vi "Live_Example_IMAQ.vi"() -> ()   [LabVIEW 2019]
doc: "This example demonstrates the image acquisition with one camera in ring buffer mode together with a live display of the latest images during record. After record is stopped, the images can be addressed by index.\nNote that this example will not be fail save, i.e. doesnt react on errors, just handles them forward to the end\n\nUsage:\nSelect your required image count, data format and the camera setup before you start the program.\nOnce started, the camera class will be initialized and images will be recorded and displayed automatically\nYou can stop the images by pressing stop record.\nAfter stopped, the image at the selected index will be read out\nTo finish the program click on quit application, this will force an exit of the camera class\nYou can change your required ROI after and also during the record."
uses:
  camera/Camera.lvclass
  pco.sdk/TimingControl/TimingControl.lvlib
panel:
  in  "Trigger":bool
  in  "data_format":T1(ring)=enum."Mono16"
  out "Image":T2(plugin-control)
  out "rawImage":u16[][](array[numeric])
  in  "Image Index":u32 max=9
  out "Recorded Images":u32
  in  "TriggerMode":T3(ring)
  in  "Quit":bool
  out "Error":errorcluster {"code" format="%x"}
  in  "Stop Record":bool
  out "Recording On":bool
  in  "cropY1":u64=2 min=1 max=1040 step=1
  in  "cropX1":u64=2 min=1 max=1392 step=1
  in  "cropY0":u64=1 min=1 max=1039 step=1
  in  "cropX0":u64=1 min=1 max=1391 step=1
  out "Image Height":u64
  out "Image Width":u64
  in  "dwImgCount":u32=10 caption="Required Number of Images" max=2397
  in  "Exposure Time [s]":dbl=0.010000000000000002 min=1e-06 max=60.0 step=0.001
  # "This example demonstrates the image acquisition with one camera in ring buffer mode together with a live display of the latest images during record. After record is stopped, the images can be addressed by index.\nNote that this example will not be fail save, i.e. doesnt react on errors, just handles them forward to the end\n\nUsage:\nSelect your required image count, data format and the camera setup before you start the program.\nOnce started, the camera class will be initialized and images will be recorded and displayed automatically\nYou can stop the images by pressing stop record.\nAfter stopped, the image at the selected index will be read out\nTo finish the program click on quit application, this will force an exit of the camera class\nYou can change the cropped region during or after recording."
  # "pco.labview"
  # "Camera Setup"
  # "Recording Control"
  # "Parameters for image readout"
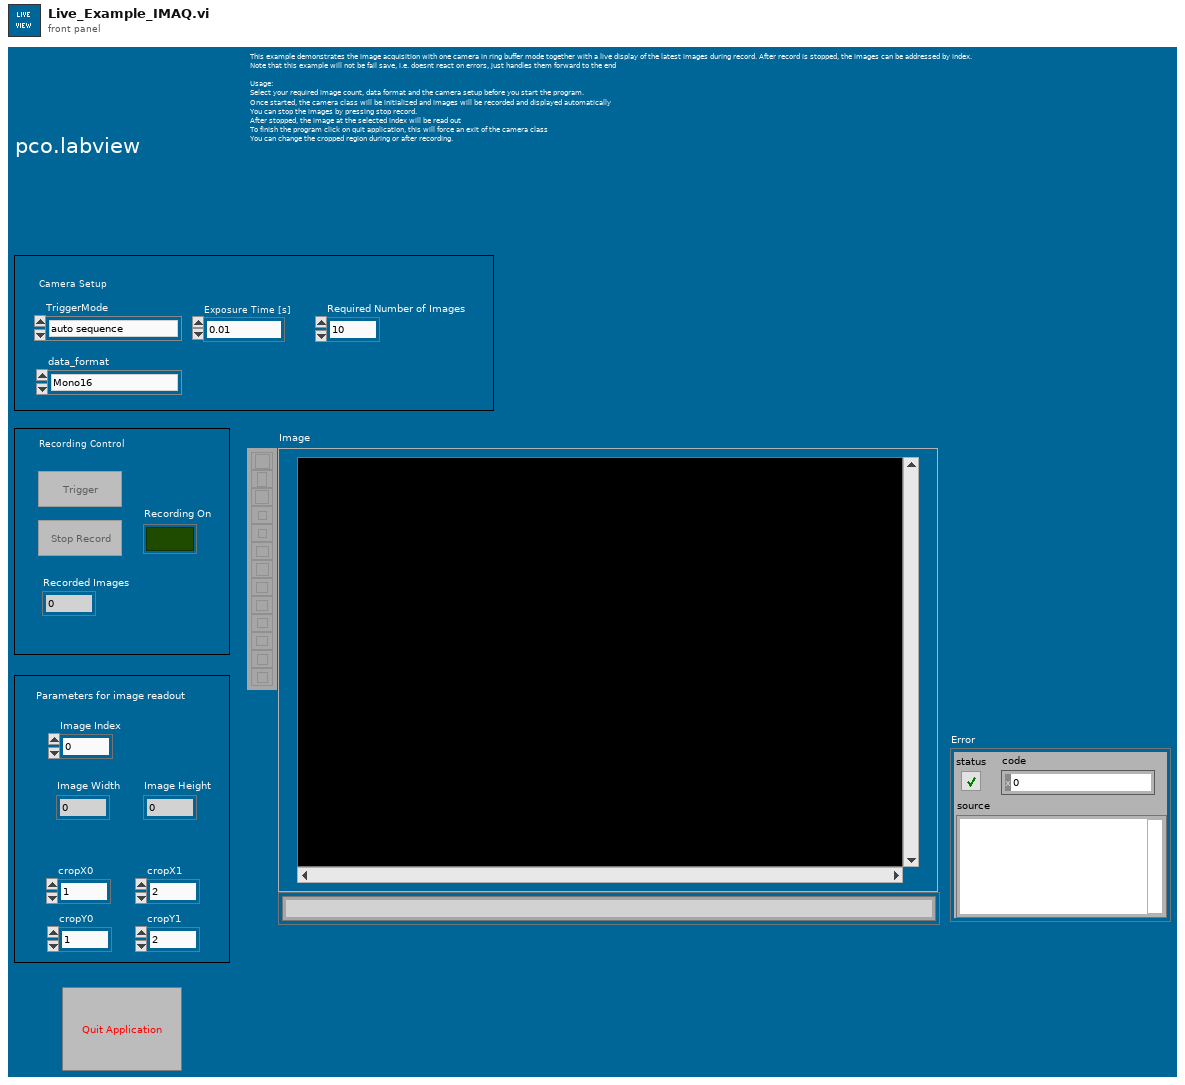
[diagram p1: front panel]
types:
  T1 = enum16{"Undefined", "Mono8", "Mono16", "BGRA8", "RGBA8", "BGRA16", "RGBA16", "CompressedMono8"}
  T2 = typedef "IMAQ Image.ctl" = refnum<image>
  T3 = enum16{"auto sequence", "software trigger", "external exposure start", "external exposure control"}
  T4 = enum16{"sequence", "sequence non blocking", "ring buffer", "fifo", "tif", "multitif", "pcoraw", "b16", "dicom", "multidicom", "camram_ring", "camram_segment"}
  T5 = enum8{"Enabled", "Disabled", "Disabled and Grayed Out"}
  T6 = cluster{"serial":u32, "type":u16, "sub_type":u16, "interface_type":u16, "bit_resolution":u16, "min_exposure_time_s":dbl, "max_exposure_time_s":dbl, "min_exposure_step_s":dbl, "min_delay_time_s":dbl, "max_delay_time_s":dbl, "min_delay_step_s":dbl, "min_width":u64, "min_height":u64, "max_width":u64, "max_height":u64, "roi_step_horz":u64, "roi_step_vert":u64, "roi_symmetric_horz":bool, "roi_symmetric_vert":bool, "has_timestamp_mode":bool, "has_timestamp_mode_ascii_only":bool, "pixelrate_vec":u32[], "conversion_factor_vec":sgl[], "has_trigger_mode_extexpctrl":bool, "has_acquire_mode":bool, "has_ext_acquire_mode":bool, "has_metadata_mode":bool, "has_ram":bool, "binning_horz_vec":u16[], "binning_vert_vec":u16[], "has_average_binning":bool, "pixel_format_vec":u32[]}
  T7 = typedef "Image Type" = u32
  T8 = cluster{"wSignalNum":u16, "wEnabled":u16, "wType":u16, "wPolarity":u16, "wFilterSetting":u16, "wSelected":u16, "dwParameter":u32[], "dwSignalFunctionality":u32[]}
  T9 = typedef "Camera.lvclass/binning.ctl" = cluster{"vert":u16, "horz":u16, "mode":u16}
  T10 = cluster{"exposure_time_s":dbl, "delay_time_s":dbl, "roi":cluster{"x0":u64, "y0":u64, "x1":u64, "y1":u64}, "timestamp_mode":u16, "pixelrate":u32, "conversion_factor":sgl, "trigger_mode":u16, "acquire_mode":u16, "acquire_sequence_number":u32, "metadata_mode":u16, "noisefilter_mode":u16, "pixel_format":u32, "binning":T9, "auto_exposure":cluster{"region":u16, "min_exposure_s":dbl, "max_exposure_s":dbl}}
  T11 = cluster{"Plane 4 (alpha)":u16, "Plane 1 (Red)":u16, "Plane 2 (Green)":u16, "Plane 3 (Blue)":u16}[][]
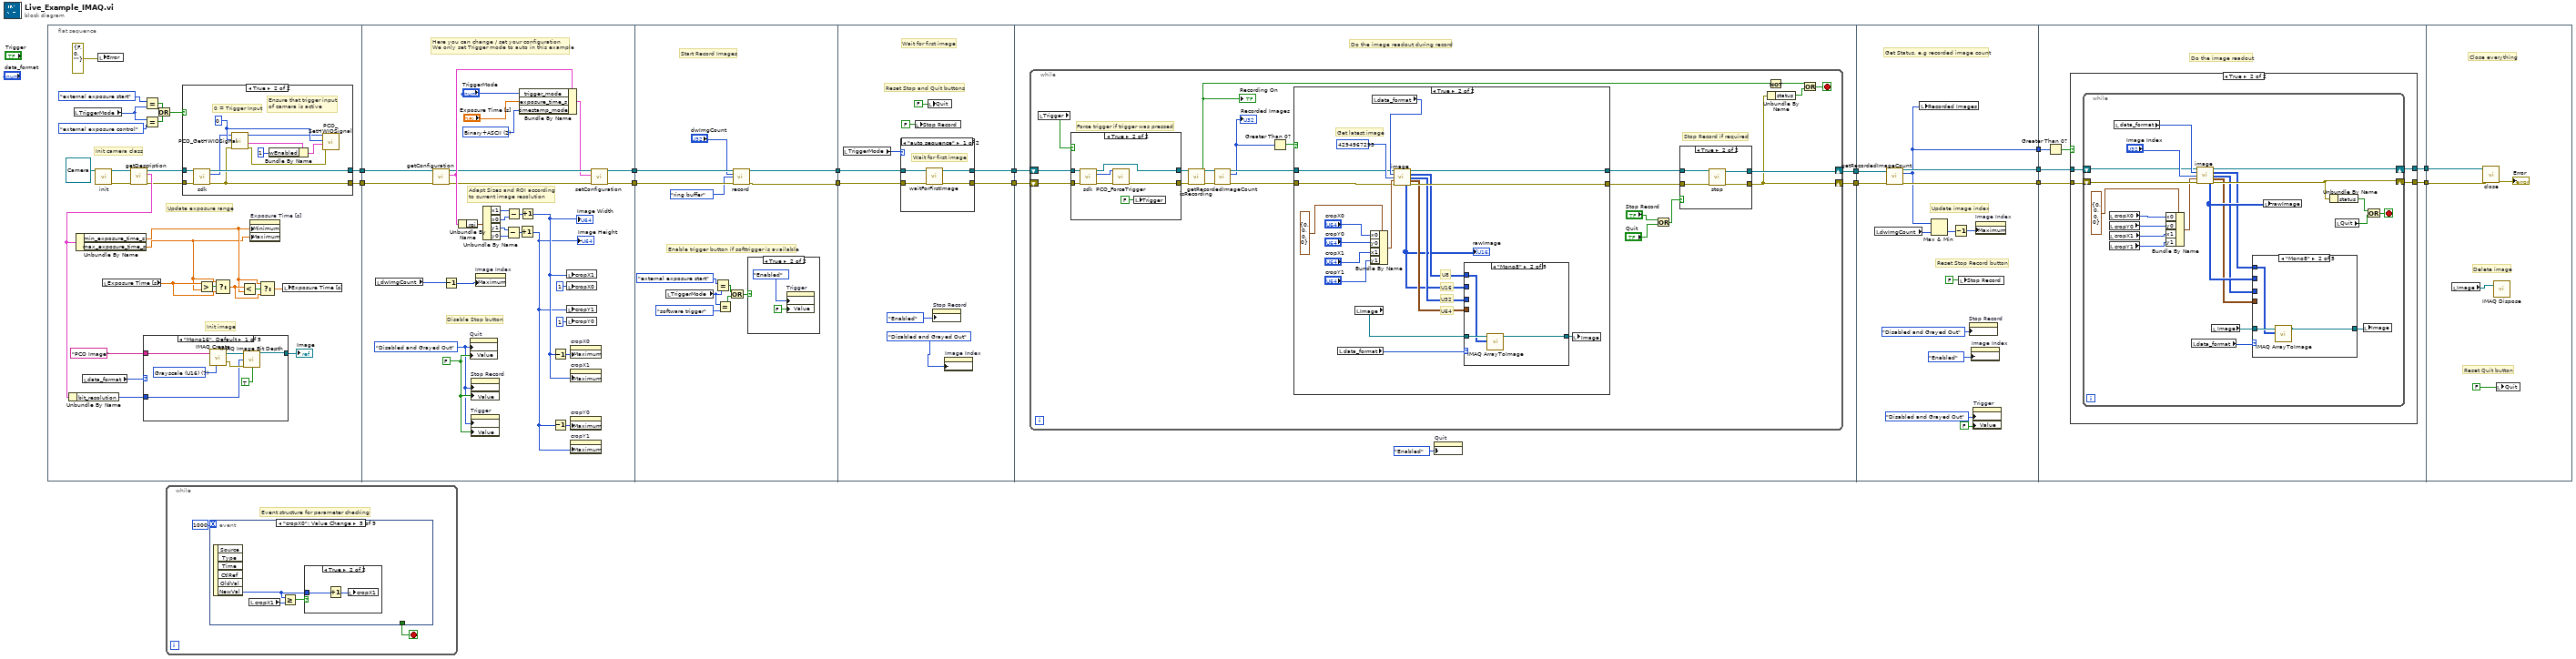
[diagram p0: block diagram]
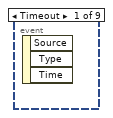
[diagram p2: hidden frame]
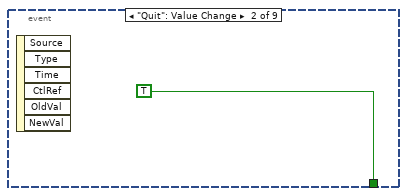
[diagram p3: hidden frame]
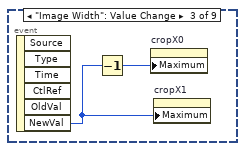
[diagram p4: hidden frame]
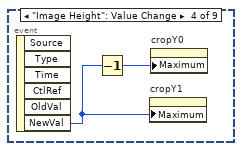
[diagram p5: hidden frame]
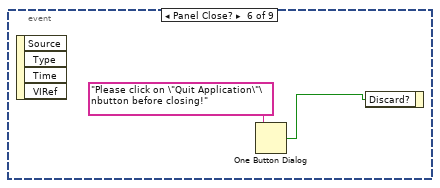
[diagram p7: hidden frame]
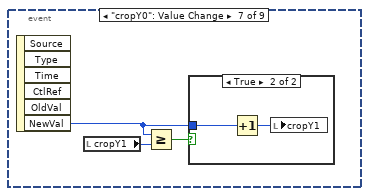
[diagram p8: hidden frame]
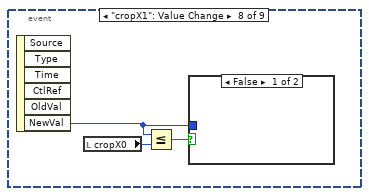
[diagram p10: hidden frame]
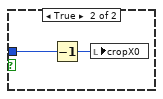
[diagram p11: hidden frame]
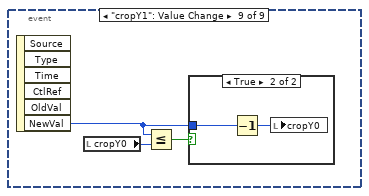
[diagram p12: hidden frame]
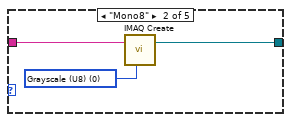
[diagram p15: hidden frame]
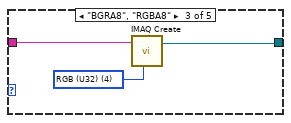
[diagram p16: hidden frame]
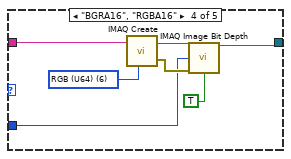
[diagram p17: hidden frame]
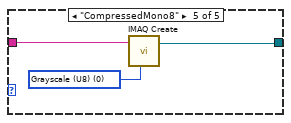
[diagram p18: hidden frame]
diagram:
  n1 = flat-sequence {
    tunnel: [w23] -> w7
    tunnel: [w22] -> w6
    tunnel: [w82] -> w15
    tunnel: [w86] -> w14
    tunnel: w7 -> [w81]
    tunnel: w6 -> [w80]
    tunnel: [w107] -> w9
    tunnel: [w108] -> w8
    tunnel: w14 -> [w117]
    tunnel: w15 -> [w116]
    tunnel: w9 -> [w124]
    tunnel: w8 -> [w125]
    tunnel: [w123] -> w13
    tunnel: [w121] -> w2
    tunnel: w13 -> [w139]
    tunnel: [w137] -> w12
    tunnel: [w136] -> w5
    tunnel: w2 -> [w135]
    tunnel: w12 -> [w222]
    tunnel: [w220] -> w11
    tunnel: w5 -> [w215]
    tunnel: [w214] -> w4
    tunnel: [w213] -> w1
    tunnel: w11 -> [w231]
    tunnel: [w230] -> w10
    tunnel: w4 -> [w229]
    tunnel: [w228] -> w3
    tunnel: w1 -> [w226]
    tunnel: w10 -> [w278]
    tunnel: w3 -> [w276]
    frame #0 {
      # "Init image"
      # "Init camera class"
      # "Update exposure range"
      n2 = local read "TriggerMode"() -> (w17:T3)
      n3 = local read "data_format"() -> (w28:T1)
      n4 = call-dynamic "init.vi"("Camera in"=refnum<class "Camera.lvclass"> refnum) -> ("Camera out"=w31:refnum<class "Camera.lvclass">, "error out"=w32:errorcluster)  [unwired: 8 in]
      n5 = local write "Error"(errorcluster {"status"=FALSE, "code"=0, "source"=""} ("error IO")) -> ()
      n6 = local read "Exposure Time [s]"() -> (w40:dbl)
      n7 = call-dynamic "getDescription.vi"("error in (no error)"=w32, "Camera in"=w31) -> ("error out"=w24:errorcluster, "description"=w27:T6, "Camera out"=w25:refnum<class "Camera.lvclass">)  [unwired: 7 in]
      n8 = Unbundle By Name(w27) -> ("bit_resolution"=w26:u16)
      n9 = Unbundle By Name(w27) -> ("min_exposure_time_s"=w30:dbl, "max_exposure_time_s"=w29:dbl)
      n10 = case shown="\"Mono16\", Default" w28 {
        tunnel: "PCO Image" ("Image Name") -> [w60 w64 w66 w73 w76]
        tunnel: [w56 w62 w65 w70 w75] -> w33
        tunnel: w26 -> [w55 _ _ w68 _]
        frame "Mono16", Default {
          w61 = T7 7 items=["Grayscale (U8)", "Grayscale (I16)", "Grayscale (SGL)", "Complex (CSG)", "RGB (U32)", "HSL (U32)", "RGB (U64)", "Grayscale (U16)"] ("Image Type")
          n11 = call "IMAQ Create"("Image Name"=w60, "Image Type"=w61) -> ("New Image"=w58:T2, "error out"=w57:errorcluster)  [unwired: 3 in]
          n12 = call "IMAQ Image Bit Depth"("Image"=w58, "Bit Depth (0)"=w55, "error in (no error)"=w57, "Get/Set Bit Depth? (Set)"=TRUE) -> ("Image Out"=w56:T2)  [unwired: 9 in, 2 out]
        }
        frame "Mono8" {
          w63 = T7 0 items=["Grayscale (U8)", "Grayscale (I16)", "Grayscale (SGL)", "Complex (CSG)", "RGB (U32)", "HSL (U32)", "RGB (U64)", "Grayscale (U16)"] ("Image Type")
          n13 = call "IMAQ Create"("Image Name"=w64, "Image Type"=w63) -> ("New Image"=w62:T2)  [unwired: 3 in, 1 out]
        }
        frame "BGRA8", "RGBA8" {
          w67 = T7 4 items=["Grayscale (U8)", "Grayscale (I16)", "Grayscale (SGL)", "Complex (CSG)", "RGB (U32)", "HSL (U32)", "RGB (U64)", "Grayscale (U16)"] ("Image Type")
          n14 = call "IMAQ Create"("Image Name"=w66, "Image Type"=w67) -> ("New Image"=w65:T2)  [unwired: 3 in, 1 out]
        }
        frame "BGRA16", "RGBA16" {
          w74 = T7 6 items=["Grayscale (U8)", "Grayscale (I16)", "Grayscale (SGL)", "Complex (CSG)", "RGB (U32)", "HSL (U32)", "RGB (U64)", "Grayscale (U16)"] ("Image Type")
          n15 = call "IMAQ Create"("Image Name"=w73, "Image Type"=w74) -> ("New Image"=w71:T2, "error out"=w69:errorcluster)  [unwired: 3 in]
          n16 = call "IMAQ Image Bit Depth"("Image"=w71, "Bit Depth (0)"=w68, "error in (no error)"=w69, "Get/Set Bit Depth? (Set)"=TRUE) -> ("Image Out"=w70:T2)  [unwired: 9 in, 2 out]
        }
        frame "CompressedMono8" {
          w77 = T7 0 items=["Grayscale (U8)", "Grayscale (I16)", "Grayscale (SGL)", "Complex (CSG)", "RGB (U32)", "HSL (U32)", "RGB (U64)", "Grayscale (U16)"] ("Image Type")
          n17 = call "IMAQ Create"("Image Name"=w76, "Image Type"=w77) -> ("New Image"=w75:T2)  [unwired: 3 in, 1 out]
        }
      }
      "Image" <- w33
      n18 = Equal?(x=T3."external exposure start" ("TriggerMode"), y=w17) -> (x = y?=w20:bool)
      n19 = Equal?(x=w17, y=T3."external exposure control" ("TriggerMode")) -> (x = y?=w19:bool)
      n20 = Or(x=w20, y=w19) -> (x .or. y?=w18:bool)
      n21 = case shown="True" w18 {
        tunnel: w25 -> [w43 w48]
        tunnel: w24 -> [w42 w47]
        tunnel: [w43 w46] -> w23
        tunnel: [w42 w44] -> w22
        frame False {
        }
        frame True {
          w52 = u16 0 ("wSignalNum")
          # "0 = Trigger Input"
          # "Ensure that trigger input\nof camera is active"
          n22 = call-dynamic "sdk.vi"("Camera in"=w48, "error in (no error)"=w47) -> ("Camera out"=w46:refnum<class "Camera.lvclass">, "sdk"=w45:u64, "error out"=w44:errorcluster)  [unwired: 11 in]
          n23 = call "PCO_GetHWIOSignal.vi"("error in (no error)"=w44, "wSignalNum"=w52, "ph"=w45) -> ("error out"=w50:errorcluster, "strSignal"=w54:T8, "ph out"=w49:u64)  [unwired: 5 in, 1 out]
          n24 = Bundle By Name(cluster=w54, "wEnabled"=u16 1) -> (w51:T8)
          n25 = call "PCO_SetHWIOSignal.vi"("error in (no error)"=w50, "strSignal"=w51, "wSignalNum"=w52, "ph"=w49) -> ()  [unwired: 5 in, 3 out]
        }
      }
      n26 = Greater?(x=w40, y=w29) -> (0:w41:bool)
      n27 = Select(t=w29, s=w41, f=w40) -> (s? t:f=w38:dbl)
      n28 = Less?(x=w38, y=w30) -> (x < y?=w39:bool)
      n29 = property on="Exposure Time [s]" class="DigNum (strict)"("Minimum"=w30, "Maximum"=w29) -> ()  [unwired: 2 in, 2 out]
      n30 = Select(t=w30, s=w39, f=w38) -> (s? t:f=w37:dbl)
      n31 = local write "Exposure Time [s]"(w37) -> ()
    }
    frame #1 {
      w92 = u16 2 items=["OFF", "Binary", "Binary+ASCII", "ASCII"] ("wTimeStampMode")
      w79 = FALSE ("Stop")
      w78 = T5."Disabled and Grayed Out" ("Disabled")
      # "Disable Stop button"
      # "Adapt Sizes and ROI according\nto current image resolution"
      # "Here you can change / set your configuration\nWe only set Trigger mode to auto in this example"
      n32 = local read "dwImgCount"() -> (w93:u32)
      n33 = call-dynamic "getConfiguration.vi"("error in (no error)"=w80, "Camera in"=w81) -> ("error out"=w87:errorcluster, "configuration"=w98:T10, "Camera out"=w89:refnum<class "Camera.lvclass">)  [unwired: 7 in]
      n34 = Decrement(x=w93) -> (x-1=w83:u32)
      n35 = Unbundle By Name(w98) -> ("roi"=w99:cluster{"x0":u64, "y0":u64, "x1":u64, "y1":u64})
      n36 = property on="Quit" class="Bool (strict)"("DisabledEnum"=w78, "Value"=w79) -> ()  [unwired: 2 in, 2 out]
      n37 = property on="Stop Record" class="Bool (strict)"("DisabledEnum"=w78, "Value"=w79) -> ()  [unwired: 2 in, 2 out]
      n38 = property on="Trigger" class="Bool (strict)"("DisabledEnum"=w78, "Value"=w79) -> ()  [unwired: 2 in, 2 out]
      n39 = property on="Image Index" class="DigNum (strict)"("Maximum"=w83) -> ()  [unwired: 2 in, 2 out]
      n40 = Unbundle By Name(w99) -> ("x1"=w101:u64, "x0"=w100:u64, "y1"=w103:u64, "y0"=w102:u64)
      n41 = Subtract(x=w103, y=w102) -> (x-y=w105:u64)
      n42 = Subtract(x=w101, y=w100) -> (x-y=w104:u64)
      n43 = Bundle By Name(cluster=w98, "trigger_mode"="TriggerMode", "exposure_time_s"="Exposure Time [s]", "timestamp_mode"=w92) -> (w88:T10)
      n44 = Increment(x=w105) -> (x+1=w84:u64)
      "Image Height" <- w84
      n45 = Increment(x=w104) -> (x+1=w85:u64)
      "Image Width" <- w85
      n46 = Decrement(x=w85) -> (x-1=w96:u64)
      n47 = Decrement(x=w84) -> (x-1=w97:u64)
      n48 = local write "cropX1"(w85) -> ()
      n49 = local write "cropX0"(u64 1 ("roiY0")) -> ()
      n50 = local write "cropY1"(w84) -> ()
      n51 = local write "cropY0"(u64 1 ("roiY0")) -> ()
      n52 = property on="cropX0" class="DigNum (strict)"("Maximum"=w96) -> ()  [unwired: 2 in, 2 out]
      n53 = property on="cropX1" class="DigNum (strict)"("Maximum"=w85) -> ()  [unwired: 2 in, 2 out]
      n54 = property on="cropY0" class="DigNum (strict)"("Maximum"=w97) -> ()  [unwired: 2 in, 2 out]
      n55 = property on="cropY1" class="DigNum (strict)"("Maximum"=w84) -> ()  [unwired: 2 in, 2 out]
      n56 = call-dynamic "setConfiguration.vi"("error in (no error)"=w87, "configuration"=w88, "Camera in"=w89) -> ("error out"=w86:errorcluster, "Camera out"=w82:refnum<class "Camera.lvclass">)  [unwired: 7 in]
    }
    frame #2 {
      # "Enable trigger button if softtrigger is available"
      # "Start Record Images"
      n57 = local read "TriggerMode"() -> (w113:T3)
      n58 = Equal?(x=T3."external exposure start" ("TriggerMode"), y=w113) -> (x = y?=w110:bool)
      n59 = Equal?(x=w113, y=T3."software trigger" ("TriggerMode")) -> (x = y?=w109:bool)
      n60 = Or(x=w110, y=w109) -> (x .or. y?=w111:bool)
      n61 = call-dynamic "record.vi"("Camera in"=w116, "num_images"="dwImgCount", "record_mode"=T4."ring buffer", "error in (no error)"=w117) -> ("Camera out"=w108:refnum<class "Camera.lvclass">, "error out"=w107:errorcluster)  [unwired: 10 in]
      n62 = case shown="True" w111 {
        frame False {
        }
        frame True {
          n63 = property on="Trigger" class="Bool (strict)"("DisabledEnum"=T5."Enabled" ("Disabled"), "Value"=FALSE ("Trigger")) -> ()  [unwired: 2 in, 2 out]
        }
      }
    }
    frame #3 {
      # "Wait for first image"
      # "Reset Stop and Quit buttons"
      n64 = local read "TriggerMode"() -> (w120:T3)
      n65 = case shown="\"auto sequence\"" w120 {
        tunnel: w125 -> [w132 w134]
        tunnel: w124 -> [w131 w133]
        tunnel: [w130 w133] -> w123
        tunnel: [w129 w134] -> w121
        frame "auto sequence" {
          # "Wait for first image"
          n66 = call-dynamic "waitForFirstImage.vi"("error in (no error)"=w131, "Camera in"=w132) -> ("error out"=w130:errorcluster, "Camera out"=w129:refnum<class "Camera.lvclass">)  [unwired: 8 in]
        }
        frame Default {
        }
      }
      n67 = local write "Stop Record"(FALSE ("Stop Record")) -> ()
      n68 = local write "Quit"(FALSE ("Stop")) -> ()
      n69 = property on="Stop Record" class="Bool (strict)"("DisabledEnum"=T5."Enabled" ("Disabled")) -> ()  [unwired: 2 in, 2 out]
      n70 = property on="Image Index" class="DigNum (strict)"("DisabledEnum"=T5."Disabled and Grayed Out" ("Disabled")) -> ()  [unwired: 2 in, 2 out]
    }
    frame #4 {
      # "Do the image readout during record"
      n71 = while {
        shift-right: [w142] -> w137
        shift-left: w139 -> [w146]
        shift-right: [w143] -> w136
        shift-left: w135 -> [w147]
        stop <- w158 stop-if-true
        # "Force trigger if trigger was pressed"
        # "Stop Record if required"
        n72 = local read "Trigger"() -> (w148:bool)
        n73 = case shown="True" w148 {
          tunnel: w147 -> [w199 w204]
          tunnel: w146 -> [w198 w203]
          tunnel: [w199 w202] -> w145
          tunnel: [w198 w201] -> w144
          frame False {
          }
          frame True {
            n74 = call-dynamic "sdk.vi"("Camera in"=w204, "error in (no error)"=w203) -> ("Camera out"=w202:refnum<class "Camera.lvclass">, "sdk"=w205:u64, "error out"=w206:errorcluster)  [unwired: 11 in]
            n75 = call "PCO_ForceTrigger.vi"("error in (no error)"=w206, "ph"=w205) -> ("error out"=w201:errorcluster)  [unwired: 6 in, 3 out]
            n76 = local write "Trigger"(FALSE ("Trigger")) -> ()
          }
        }
        n77 = call-dynamic "isRecording.vi"("Camera in"=w145, "error in (no error)"=w144) -> ("Camera out"=w153:refnum<class "Camera.lvclass">, "recording"=w156:bool, "error out"=w152:errorcluster)  [unwired: 11 in]
        "Recording On" <- w156
        n78 = call-dynamic "getRecordedImageCount.vi"("Camera in"=w153, "error in (no error)"=w152) -> ("Camera out"=w150:refnum<class "Camera.lvclass">, "recorded_image_count"=w140:u32, "error out"=w151:errorcluster)  [unwired: 11 in]
        "Recorded Images" <- w140
        n79 = Greater Than 0?(x=w140) -> (x > 0?=w141:bool)
        n80 = case shown="True" w141 {
          tunnel: [w162 w177] -> w154
          tunnel: w151 -> [w162 w174]
          tunnel: w150 -> [w163 w165]
          tunnel: [w163 w164] -> w149
          frame False {
          }
          frame True {
            # "U64"
            # "U32"
            # "U8"
            # "U16"
            # "Get latest image"
            n81 = local read "data_format"() -> (w166:T1)
            n82 = local read "Image"() -> (w171:T2)
            n83 = Bundle By Name(cluster=cluster{"x0":u64, "y0":u64, "x1":u64, "y1":u64} {"x0"=0, "y0"=0, "x1"=0, "y1"=0} ("roi"), "x0"="cropX0", "y0"="cropY0", "x1"="cropX1", "y1"="cropY1") -> (w178:cluster{"x0":u64, "y0":u64, "x1":u64, "y1":u64})
            n84 = local read "data_format"() -> (w173:T1)
            n85 = call-dynamic "image.vi"("Camera in"=w165, "data_format"=w173, "image_index"=u32 4294967295 ("dwImgIdx"), "crop"=w178, "error in (no error)"=w174) -> ("Camera out"=w164:refnum<class "Camera.lvclass">, "image (U8)"=w168:u8[][], "image (U32)"=w169:u32[][], "image (U64)"=w170:T11, "raw_image (U16)"=w167:u16[][], "error out"=w177:errorcluster)  [unwired: 2 in, 3 out]
            "rawImage" <- w167
            n86 = case shown="\"Mono8\"" w166 {
              tunnel: w171 -> [w185 w188 w191 w194 w197]
              tunnel: [w183 w186 w190 w192 w196] -> w172
              tunnel: w170 -> [_ _ _ w193 _]
              tunnel: w169 -> [_ _ w189 _ _]
              tunnel: w168 -> [_ w187 _ _ w195]
              tunnel: w167 -> [w184 _ _ _ _]
              frame "Mono16", Default {
                n87 = call "IMAQ ArrayToImage"("Image Pixels (U16)"=w184, "Image"=w185) -> ("Image Out"=w183:T2)  [unwired: 8 in, 1 out]
              }
              frame "Mono8" {
                n88 = call "IMAQ ArrayToImage"("Image Pixels (U8)"=w187, "Image"=w188) -> ("Image Out"=w186:T2)  [unwired: 8 in, 1 out]
              }
              frame "BGRA8", "RGBA8" {
                n89 = call "IMAQ ArrayToColorImage"("Image Pixels (U32)"=w189, "Image"=w191) -> ("Image Out"=w190:T2)  [unwired: 3 in, 1 out]
              }
              frame "BGRA16", "RGBA16" {
                n90 = call "IMAQ ArrayToColorImage"("Image"=w194, "Image Pixels (U64)"=w193) -> ("Image Out"=w192:T2)  [unwired: 3 in, 1 out]
              }
              frame "CompressedMono8" {
                n91 = call "IMAQ ArrayToImage"("Image Pixels (U8)"=w195, "Image"=w197) -> ("Image Out"=w196:T2)  [unwired: 8 in, 1 out]
              }
            }
            n92 = local write "Image"(w172) -> ()
          }
        }
        n93 = Or(x="Stop Record", y="Quit") -> (x .or. y?=w159:bool)
        n94 = case shown="True" w159 {
          tunnel: w154 -> [w208 w209]
          tunnel: [w207 w211] -> w143
          tunnel: [w208 w212] -> w142
          tunnel: w149 -> [w207 w210]
          frame False {
          }
          frame True {
            n95 = call-dynamic "stop.vi"("error in (no error)"=w209, "Camera in"=w210) -> ("error out"=w212:errorcluster, "Camera out"=w211:refnum<class "Camera.lvclass">)  [unwired: 8 in]
          }
        }
        n96 = Unbundle By Name(w142) -> ("status"=w157:bool)
        n97 = Not(x=w156) -> (.not. x?=w155:bool)
        n98 = Or(x=w155, y=w157) -> (x .or. y?=w158:bool)
      }
      n99 = property on="Quit" class="Bool (strict)"("DisabledEnum"=T5."Enabled" ("Disabled")) -> ()  [unwired: 2 in, 2 out]
    }
    frame #5 {
      # "Update image index"
      # "Reset Stop Record button"
      # "Get Status, e.g recorded image count"
      n100 = local read "dwImgCount"() -> (w221:u32)
      n101 = call-dynamic "getRecordedImageCount.vi"("Camera in"=w215, "error in (no error)"=w222) -> ("Camera out"=w214:refnum<class "Camera.lvclass">, "recorded_image_count"=w213:u32, "error out"=w220:errorcluster)  [unwired: 11 in]
      n102 = local write "Recorded Images"(w213) -> ()
      n103 = Max & Min(x=w213, y=w221) -> (min(x,y)=w223:u32)  [unwired: 1 out]
      n104 = Decrement(x=w223) -> (x-1=w218:u32)
      n105 = local write "Stop Record"(FALSE ("Stop Record")) -> ()
      n106 = property on="Stop Record" class="Bool (strict)"("DisabledEnum"=T5."Disabled and Grayed Out" ("Disabled")) -> ()  [unwired: 2 in, 2 out]
      n107 = property on="Image Index" class="DigNum (strict)"("DisabledEnum"=T5."Enabled" ("Disabled")) -> ()  [unwired: 2 in, 2 out]
      n108 = property on="Trigger" class="Bool (strict)"("DisabledEnum"=T5."Disabled and Grayed Out" ("Disabled"), "Value"=FALSE ("Trigger")) -> ()  [unwired: 2 in, 2 out]
      n109 = property on="Image Index" class="DigNum (strict)"("Maximum"=w218) -> ()  [unwired: 2 in, 2 out]
    }
    frame #6 {
      # "Do the image readout"
      n110 = Greater Than 0?(x=w226) -> (x > 0?=w227:bool)
      n111 = case shown="True" w227 {
        tunnel: w231 -> [w232 w237]
        tunnel: [w232 w236] -> w230
        tunnel: w229 -> [w233 w235]
        tunnel: [w233 w234] -> w228
        frame False {
        }
        frame True {
          n112 = while {
            shift-right: [w251] -> w236
            shift-left: w237 -> [w259]
            shift-right: [w238] -> w234
            shift-left: w235 -> [w239]
            stop <- w253 stop-if-true
            n113 = local read "cropX0"() -> (w249:u64)
            n114 = local read "cropY0"() -> (w250:u64)
            n115 = local read "cropX1"() -> (w257:u64)
            n116 = local read "cropY1"() -> (w256:u64)
            n117 = local read "data_format"() -> (w247:T1)
            n118 = Bundle By Name(cluster=cluster{"x0":u64, "y0":u64, "x1":u64, "y1":u64} {"x0"=0, "y0"=0, "x1"=0, "y1"=0} ("roi"), "x0"=w249, "y0"=w250, "x1"=w257, "y1"=w256) -> (w258:cluster{"x0":u64, "y0":u64, "x1":u64, "y1":u64})
            n119 = local read "data_format"() -> (w240:T1)
            n120 = call-dynamic "image.vi"("Camera in"=w239, "data_format"=w247, "image_index"="Image Index", "crop"=w258, "error in (no error)"=w259) -> ("Camera out"=w238:refnum<class "Camera.lvclass">, "image (U8)"=w243:u8[][], "image (U32)"=w242:u32[][], "image (U64)"=w241:T11, "raw_image (U16)"=w244:u16[][], "error out"=w251:errorcluster)  [unwired: 2 in, 3 out]
            n121 = local read "Image"() -> (w245:T2)
            n122 = case shown="\"Mono8\"" w240 {
              tunnel: w245 -> [w262 w265 w268 w271 w274]
              tunnel: [w260 w263 w267 w269 w273] -> w246
              tunnel: w241 -> [_ _ _ w270 _]
              tunnel: w242 -> [_ _ w266 _ _]
              tunnel: w243 -> [_ w264 _ _ w272]
              tunnel: w244 -> [w261 _ _ _ _]
              frame "Mono16", Default {
                n123 = call "IMAQ ArrayToImage"("Image Pixels (U16)"=w261, "Image"=w262) -> ("Image Out"=w260:T2)  [unwired: 8 in, 1 out]
              }
              frame "Mono8" {
                n124 = call "IMAQ ArrayToImage"("Image Pixels (U8)"=w264, "Image"=w265) -> ("Image Out"=w263:T2)  [unwired: 8 in, 1 out]
              }
              frame "BGRA8", "RGBA8" {
                n125 = call "IMAQ ArrayToColorImage"("Image Pixels (U32)"=w266, "Image"=w268) -> ("Image Out"=w267:T2)  [unwired: 3 in, 1 out]
              }
              frame "BGRA16", "RGBA16" {
                n126 = call "IMAQ ArrayToColorImage"("Image"=w271, "Image Pixels (U64)"=w270) -> ("Image Out"=w269:T2)  [unwired: 3 in, 1 out]
              }
              frame "CompressedMono8" {
                n127 = call "IMAQ ArrayToImage"("Image Pixels (U8)"=w272, "Image"=w274) -> ("Image Out"=w273:T2)  [unwired: 8 in, 1 out]
              }
            }
            n128 = local write "rawImage"(w244) -> ()
            n129 = Unbundle By Name(w251) -> ("status"=w254:bool)
            n130 = local read "Quit"() -> (w255:bool)
            n131 = local write "Image"(w246) -> ()
            n132 = Or(x=w254, y=w255) -> (x .or. y?=w253:bool)
          }
        }
      }
    }
    frame #7 {
      # "Delete image"
      # "Close everything"
      # "Reset Quit button"
      n133 = local read "Image"() -> (w275:T2)
      n134 = call-dynamic "close.vi"("error in (no error)"=w278, "Camera in"=w276) -> ("error out"=→"Error":errorcluster)  [unwired: 9 in]
      n135 = call "IMAQ Dispose"("Image"=w275) -> ()  [unwired: 5 in, 1 out]
      n136 = local write "Quit"(FALSE ("Stop Record")) -> ()
    }
  }
  n137 = while {
    stop <- w280 stop-if-true
    # "Event structure for parameter checking"
    n138 = event shown="[4] \"cropX0\": Value Change" {
      selector: _ -> [_ _ _ _ _ _ _ _ _]
      dyn-events: _ -> [_ _ _ _ _ _ _ _ _]
      timeout: 1000 -> [_ _ _ _ _ _ _ _ _]
      tunnel: [_ TRUE _ _ _ _ _ _ _] -> w280
      event Timeout {
        n139 = event-data() -> ()  [unwired: 1 in, 3 out]
      }
      event "Quit": Value Change {
        n140 = event-data() -> ()  [unwired: 1 in, 6 out]
      }
      event "Image Width": Value Change {
        n141 = event-data() -> ("NewVal"=w283:u64)  [unwired: 1 in, 5 out]
        n142 = Decrement(x=w283) -> (x-1=w284:u64)
        n143 = property on="cropX0" class="DigNum (strict)"("Maximum"=w284) -> ()  [unwired: 2 in, 2 out]
        n144 = property on="cropX1" class="DigNum (strict)"("Maximum"=w283) -> ()  [unwired: 2 in, 2 out]
      }
      event "Image Height": Value Change {
        n145 = event-data() -> ("NewVal"=w285:u64)  [unwired: 1 in, 5 out]
        n146 = Decrement(x=w285) -> (x-1=w286:u64)
        n147 = property on="cropY1" class="DigNum (strict)"("Maximum"=w285) -> ()  [unwired: 2 in, 2 out]
        n148 = property on="cropY0" class="DigNum (strict)"("Maximum"=w286) -> ()  [unwired: 2 in, 2 out]
      }
      event "cropX0": Value Change {
        n149 = event-data() -> ("NewVal"=w287:u64)  [unwired: 1 in, 5 out]
        n150 = local read "cropX1"() -> (w289:u64)
        n151 = Greater Or Equal?(x=w287, y=w289) -> (x >= y?=w288:bool)
        n152 = case shown="True" w288 {
          tunnel: w287 -> [_ w291]
          frame False {
          }
          frame True {
            n153 = Increment(x=w291) -> (x+1=w290:u64)
            n154 = local write "cropX1"(w290) -> ()
          }
        }
      }
      event Panel Close? {
        n155 = event-data() -> ()  [unwired: 1 in, 4 out]
        n156 = One Button Dialog(message="Please click on \"Quit Application\"\nbutton before closing!") -> (true=w292:bool)  [unwired: 1 in]
        n157 = event-data("Discard?"=w292) -> ()  [unwired: 1 in, 1 out]
      }
      event "cropY0": Value Change {
        n158 = event-data() -> ("NewVal"=w294:u64)  [unwired: 1 in, 5 out]
        n159 = local read "cropY1"() -> (w296:u64)
        n160 = Greater Or Equal?(x=w294, y=w296) -> (x >= y?=w295:bool)
        n161 = case shown="True" w295 {
          tunnel: w294 -> [_ w298]
          frame False {
          }
          frame True {
            n162 = Increment(x=w298) -> (x+1=w297:u64)
            n163 = local write "cropY1"(w297) -> ()
          }
        }
      }
      event "cropX1": Value Change {
        n164 = event-data() -> ("NewVal"=w299:u64)  [unwired: 1 in, 5 out]
        n165 = local read "cropX0"() -> (w301:u64)
        n166 = Less Or Equal?(x=w299, y=w301) -> (x <= y?=w300:bool)
        n167 = case shown="False" w300 {
          tunnel: w299 -> [_ w303]
          frame False {
          }
          frame True {
            n168 = Decrement(x=w303) -> (x-1=w302:u64)
            n169 = local write "cropX0"(w302) -> ()
          }
        }
      }
      event "cropY1": Value Change {
        n170 = event-data() -> ("NewVal"=w304:u64)  [unwired: 1 in, 5 out]
        n171 = local read "cropY0"() -> (w306:u64)
        n172 = Less Or Equal?(x=w304, y=w306) -> (x <= y?=w305:bool)
        n173 = case shown="True" w305 {
          tunnel: w304 -> [_ w308]
          frame False {
          }
          frame True {
            n174 = Decrement(x=w308) -> (x-1=w307:u64)
            n175 = local write "cropY0"(w307) -> ()
          }
        }
      }
    }
  }
